vi "Test Old Report is Not Overwritten on Seconde Test Start.vi"(8 "error in (no error)":errorcluster, 11 "XML Report Test in":refnum<class "Report Generator Test.lvclass">) -> (0 "error out":errorcluster, 3 "XML Report Test out":refnum<class "Report Generator Test.lvclass">)   [LabVIEW 2020, in "Report Generator Test.lvclass"]
uses:
  Report Generator Test.lvclass
  C:/Program Files (x86)/National Instruments/LabVIEW 2020/vi.lib/Astemes/LUnit/Core/LUnit Test Case/Test Case.lvclass
  Report Generator Test.lvclass/Report Generator Test.ctl
  <vilib>/Astemes/LUnit/Core/LUnit Test Case/Test Case.lvclass/Test Case.ctl
  538b6b46-2778-4cbc-9a22-6f9245e30f78.vi
  <vilib>/Astemes/LUnit/Core/LUnit Test Case/Private/Append Fail Result.vi
  <vilib>/Astemes/LUnit/Core/LUnit Test Case/Private/Append Pass Result.vi
  538b6b46-2778-4cbc-9a22-6f9245e30f78.vi/4479f1b4-f4e5-41cd-8a07-3589632eefcf.vi
  <vilib>/Astemes/LUnit/Core/LUnit Test Case/Private/Run In UI.vi
  Test Doubles/Mock Report/Mock Report.lvclass
  C:/git/astemes-lunit/source/Plugins/Report/Report.lvclass
  source/Plugins/Report/Report.lvclass
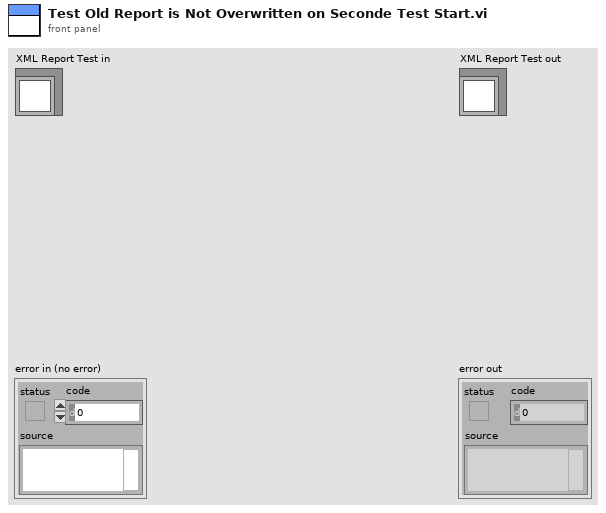
[diagram p1: front panel]
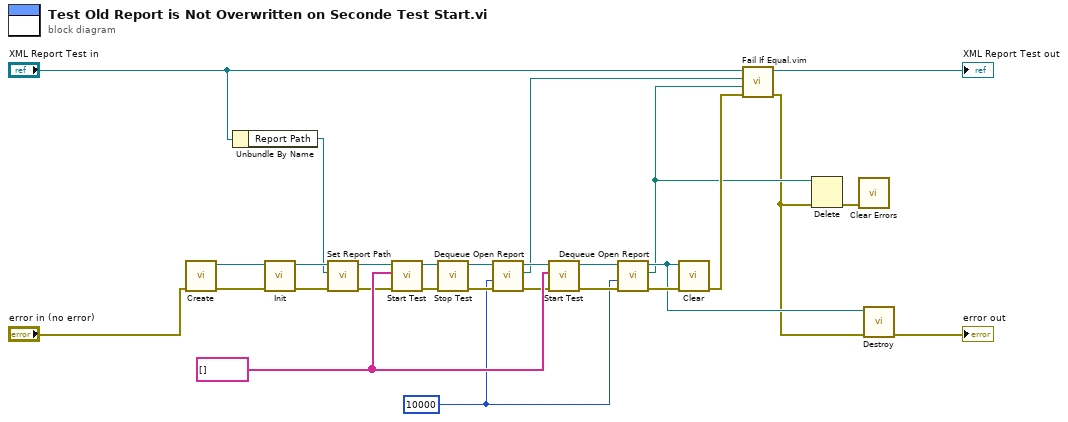
[diagram p0: block diagram]
diagram:
  w4 = 10000 ("timeout in ms (0)")
  w14 = string[] [] ("Tests")
  n1 = call "Create.vi"("error in (no error)"="error in (no error)") -> ("error out"=w21:errorcluster, "Mock Report Out"=w23:refnum<class "Mock Report.lvclass">)  [unwired: 9 in]
  n2 = Unbundle By Name("XML Report Test in") -> ("Report Path"=w6:path)
  n3 = call-dynamic "Init.vi"("error in (no error)"=w21, "Mock Report In"=w23) -> ("error out"=w27:errorcluster, "Mock Report Out"=w9:refnum<class "Mock Report.lvclass">)  [unwired: 8 in]
  n4 = call "Set Report Path.vi"("error in (no error)"=w27, "Report Path"=w6, "Report In"=w9) -> ("error out"=w10:errorcluster, "Report Out"=w8:refnum<class "Mock Report.lvclass">)  [unwired: 7 in]
  n5 = call-dynamic "Start Test.vi"("error in (no error)"=w10, "Tests"=w14, "XML Report in"=w8) -> ("error out"=w26:errorcluster, "XML Report out"=w17:refnum<class "Mock Report.lvclass">)  [unwired: 7 in]
  n6 = call-dynamic "Stop Test.vi"("error in (no error)"=w26, "XML Report in"=w17) -> ("error out"=w18:errorcluster, "XML Report out"=w12:refnum<class "Mock Report.lvclass">)  [unwired: 8 in]
  n7 = call "Dequeue Open Report.vi"("error in (no error)"=w18, "timeout in ms (0)"=w4, "Mock Report In"=w12) -> ("error out"=w13:errorcluster, "path"=w5:path, "Mock Report Out"=w11:refnum<class "Mock Report.lvclass">)  [unwired: 5 in, 1 out]
  n8 = call-dynamic "Start Test.vi"("error in (no error)"=w13, "Tests"=w14, "XML Report in"=w11) -> ("error out"=w16:errorcluster, "XML Report out"=w15:refnum<class "Mock Report.lvclass">)  [unwired: 7 in]
  n9 = call "Dequeue Open Report.vi"("error in (no error)"=w16, "timeout in ms (0)"=w4, "Mock Report In"=w15) -> ("error out"=w25:errorcluster, "path"=w3:path, "Mock Report Out"=w19:refnum<class "Mock Report.lvclass">)  [unwired: 5 in, 1 out]
  n10 = call-dynamic "Clear.vi"("error in (no error)"=w25, "XML Report in"=w19) -> ("error out"=w24:errorcluster)  [unwired: 9 in]
  n11 = call "Fail If Equal.vim"("error in (no error)"=w24, "Actual"=w3, "Unexpected"=w5, "LUnit Test Case In"="XML Report Test in") -> ("error out"=w2:errorcluster, "LUnit Test Case Out"=→"XML Report Test out":refnum<class "Report Generator Test.lvclass">)  [unwired: 6 in]
  n12 = Delete(path (use dialog)=w3, error in=w2) -> (error out=w1:errorcluster)  [unwired: 3 in, 2 out]
  n13 = call <vilib>:"Clear Errors.vi"("error in (no error)"=w1) -> ()  [unwired: 5 in, 2 out]
  n14 = call "Destroy.vi"("error in (no error)"=w2, "Mock Report In"=w19) -> ("error out"=→"error out":errorcluster)  [unwired: 9 in]
